vi "3. NumericOps.vi"() -> ()   [LabVIEW 2019]
panel:
  out "Div":dbl
  out "Mult":dbl
  out "Sub":dbl
  out "Sum":dbl
  in  "Num2":dbl
  in  "Num1":dbl
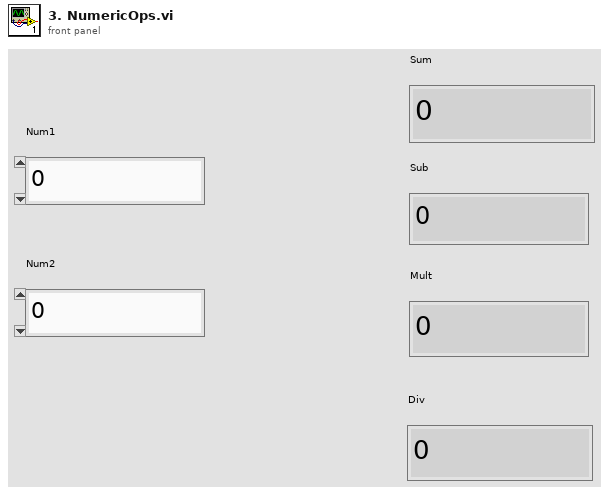
[diagram p1: front panel]
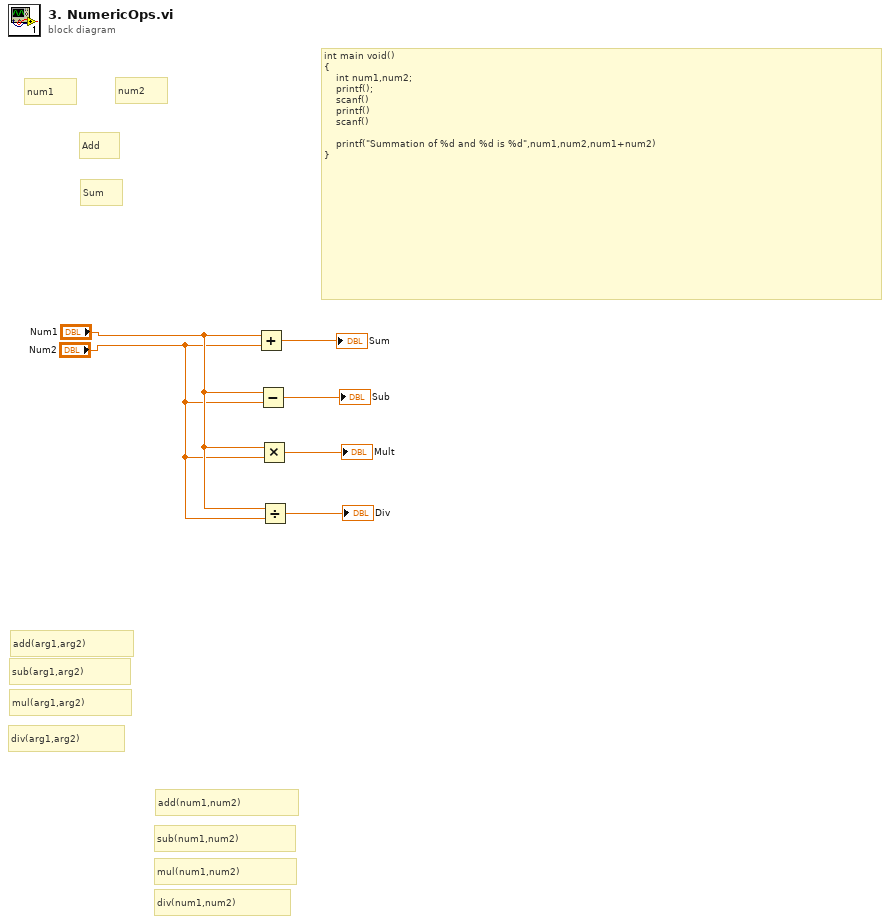
[diagram p0: block diagram]
diagram:
  # "div(num1,num2)"
  # "mul(num1,num2)"
  # "sub(num1,num2)"
  # "add(num1,num2)"
  # "div(arg1,arg2)"
  # "mul(arg1,arg2)"
  # "sub(arg1,arg2)"
  # "add(arg1,arg2)"
  # "Sum"
  # "Add"
  # "num2"
  # "num1"
  # "int main void()\n{\n    int num1,num2;\n    printf();\n    scanf()\n    printf()\n    scanf()\n   \n    printf(\"Summation of %d and %d is %d\",num1,num2,num1+num2)\n}"
  n1 = Add(x="Num1", y="Num2") -> (x+y=→"Sum":dbl)
  n2 = Subtract(x="Num1", y="Num2") -> (x-y=→"Sub":dbl)
  n3 = Multiply(x="Num1", y="Num2") -> (x*y=→"Mult":dbl)
  n4 = Divide(x="Num1", y="Num2") -> (x/y=→"Div":dbl)
